vi "SaveFiles.vi"(0 "Refnum in":refnum<k34>, 1 "Analyte":string, 2 "fileCreateTime":timestamp, 4 "Array 2":waveform(dbl)[](array[waveform]), 6 "ParameterValues":string[](array[string]), 8 "output path":path, 10 "ParameterNames":string[](array[string])) -> (14 "Refnum out":refnum<k34>, 15 "seconds since 1Jan1904":timestamp)   [LabVIEW 2024]
panel:
  out "error out":errorcluster
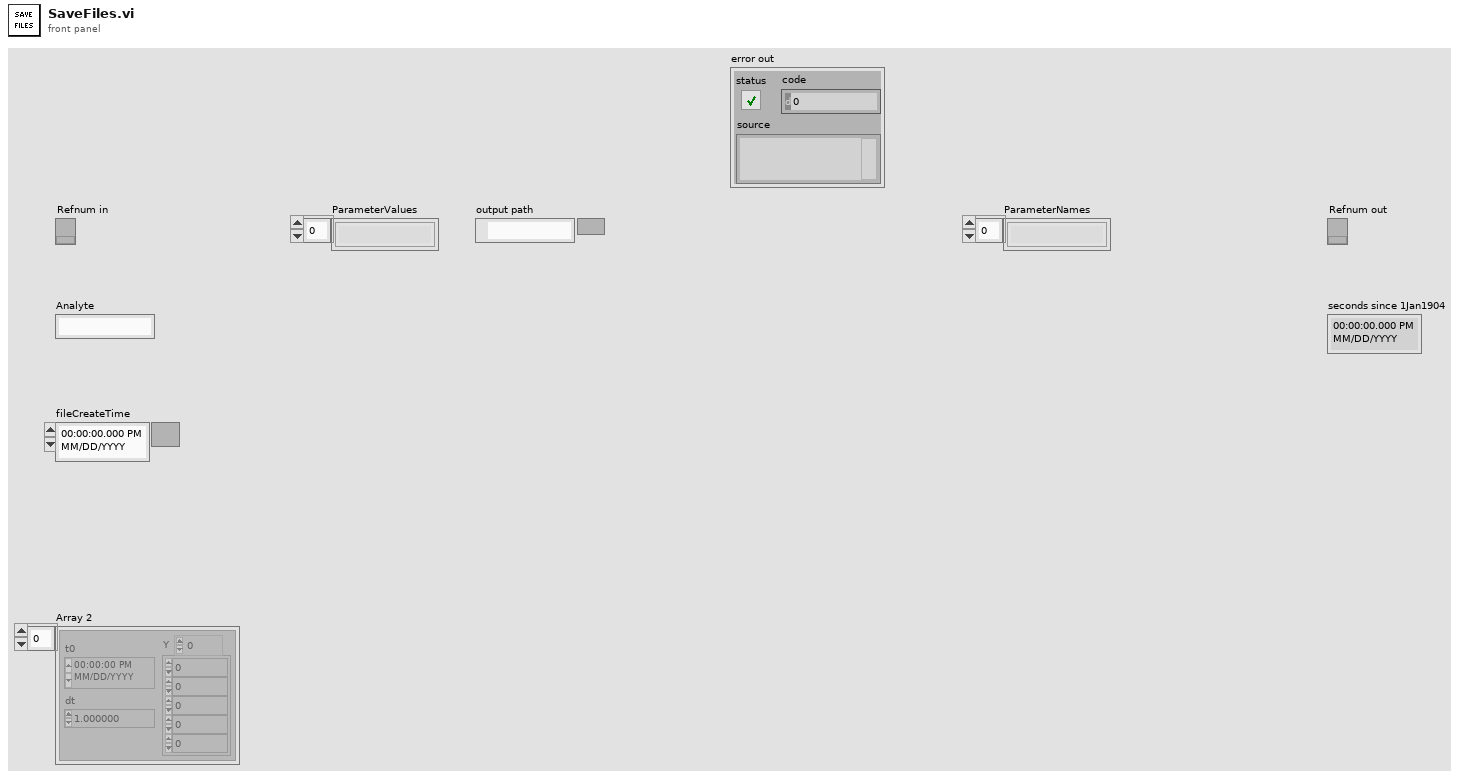
[diagram p1: front panel]
types:
  T1 = enum16{"open", "open or create", "create or replace", "create", "open (read-only)"}
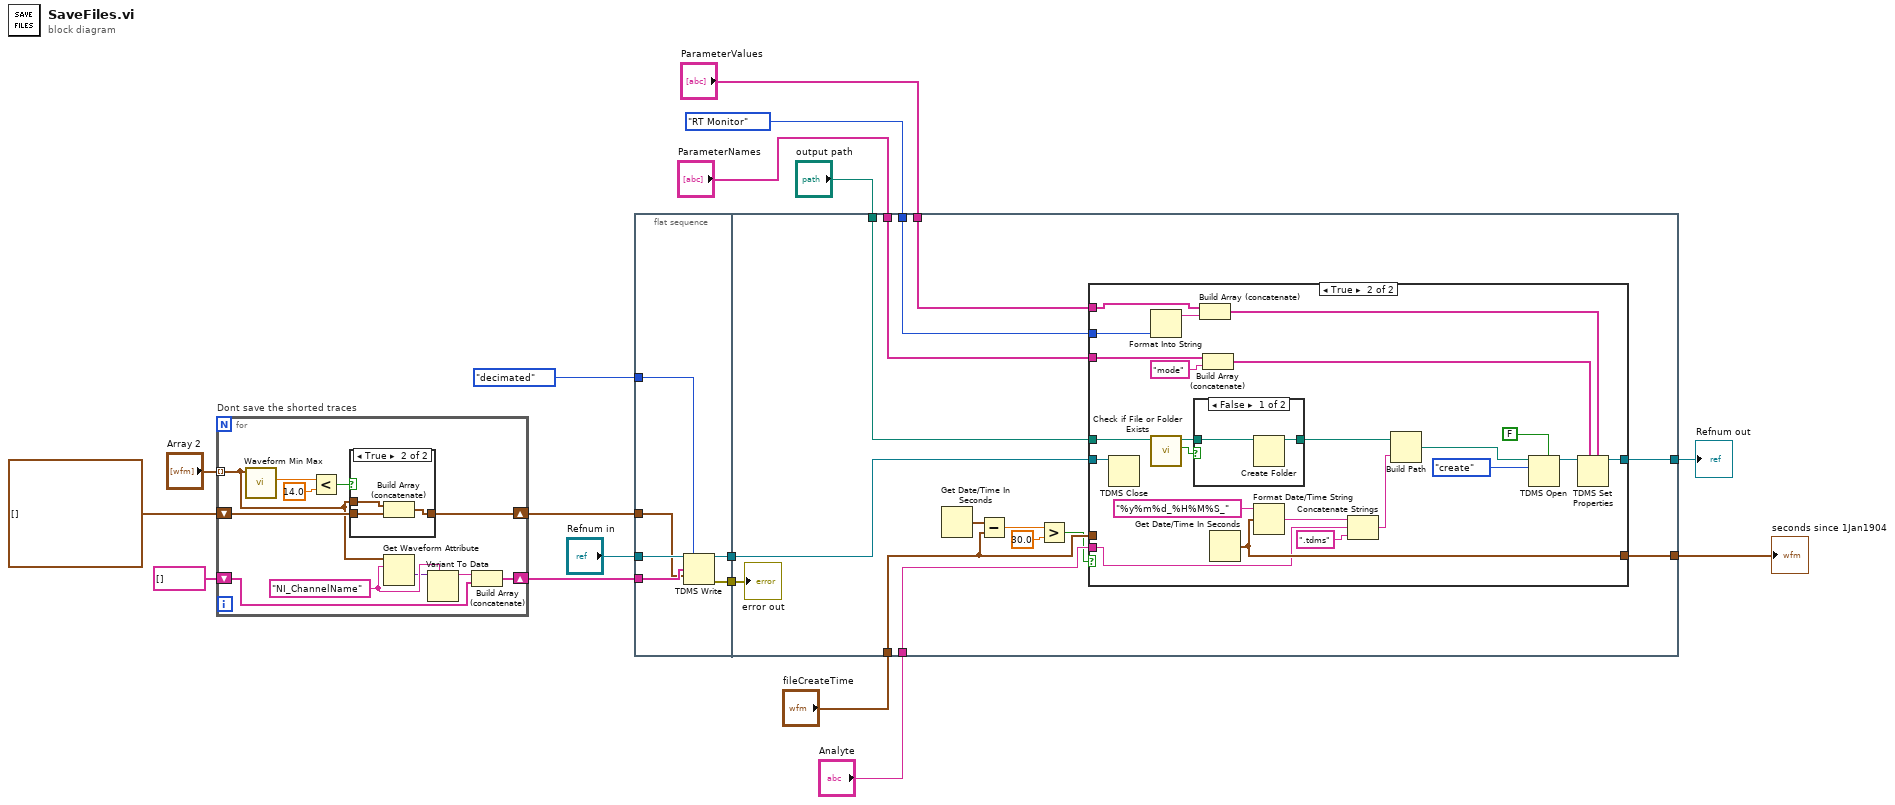
[diagram p0: block diagram]
diagram:
  n1 = for "Dont save the shorted traces" {
    tunnel: "Array 2" -> [w19] mode=indexing
    shift-right: [w25] -> w10
    shift-left: waveform(dbl)[] [] -> [w26]
    shift-right: [w24] -> w9
    shift-left: string[] [] -> [w23]
    w22 = "NI_ChannelName" ("name")
    n2 = call <vilib>:"Waveform Min Max.vi"("waveform in"=w19) -> ("Y max"=w18:dbl)  [unwired: 5 in, 5 out]
    n3 = Less?(x=w18, y=14.0) -> (x < y?=w27:bool)
    n4 = case shown="True" w27 {
      tunnel: w19 -> [_ w32]
      tunnel: [w29 w31] -> w25
      tunnel: w26 -> [w29 w30]
      frame False {
      }
      frame True {
        n5 = Build Array (concatenate)(w32, w30) -> (w31:waveform(dbl)[])
      }
    }
    n6 = Get Waveform Attribute(6:w22, 7:w19) -> (1:w20:variant)  [unwired: 2 in, 3 out]
    n7 = Variant To Data(type=w22, Variant=w20) -> (data=w21:string)  [unwired: 1 in, 1 out]
    n8 = Build Array (concatenate)(w21, w23) -> (w24:string[])
  }
  n9 = flat-sequence {
    tunnel: "Refnum in" -> [w38]
    tunnel: enum16{"decimated", "interleaved"}."decimated" ("data layout (0:decimated)") -> [w37]
    tunnel: w9 -> [w36]
    tunnel: w10 -> [w35]
    tunnel: [w34] -> w2
    tunnel: [w33] -> w1
    tunnel: w2 -> [w52]
    tunnel: enum32{"RT Monitor", "IV Monitor"}."RT Monitor" ("Value") -> [w51]
    tunnel: [w50] -> w11
    tunnel: [w49] -> w12
    tunnel: "fileCreateTime" -> [w44]
    tunnel: "output path" -> [w48]
    tunnel: "ParameterNames" -> [w47]
    tunnel: "ParameterValues" -> [w46]
    tunnel: "Analyte" -> [w45]
    tunnel: w1 -> [w39]
    frame #0 {
      n10 = TDMS Write(0:w38, 1:w37, 7:w36, 9:w35) -> (4:w34:refnum<k34>, 15:w33:errorcluster)  [unwired: 2 in, 2 out]
    }
    frame #1 {
      n11 = Get Date/Time In Seconds() -> (seconds since 1Jan1904=w42:timestamp)
      n12 = Subtract(x=w42, y=w44) -> (x-y=w43:dbl)
      n13 = Greater?(x=w43, y=30.0) -> (0:w40:bool)
      n14 = case shown="True" w40 {
        tunnel: w52 -> [w54 w63]
        tunnel: w51 -> [_ w62]
        tunnel: [w54 w60] -> w50
        tunnel: [w53 w59] -> w49
        tunnel: w48 -> [_ w58]
        tunnel: w47 -> [_ w57]
        tunnel: w46 -> [_ w56]
        tunnel: w45 -> [_ w55]
        tunnel: w44 -> [w53 _]
        frame False {
        }
        frame True {
          n15 = TDMS Close(11:w63) -> ()  [unwired: 1 in, 2 out]
          n16 = Format Into String(w62) -> (resulting string=w61:string)  [unwired: 3 in, 1 out]
          n17 = call <vilib>:"Check if File or Folder Exists.vi"("path"=w58) -> ("file or folder exists?"=w77:bool, "dup path"=w72:path)  [unwired: 8 in, 1 out]
          n18 = case shown="False" w77 {
            tunnel: w72 -> [w79 w80]
            tunnel: [w78 w80] -> w73
            frame False {
              n19 = Create Folder(path (use dialog)=w79) -> (created path=w78:path)  [unwired: 2 in, 2 out]
            }
            frame True {
            }
          }
          n20 = Build Array (concatenate)(w56, w61) -> (w65:string[])
          n21 = Build Array (concatenate)(w57, "mode") -> (w64:string[])
          n22 = Get Date/Time In Seconds() -> (seconds since 1Jan1904=w59:timestamp)
          n23 = Format Date/Time String(time format string (%c)="%y%m%d_%H%M%S_", seconds (now)=w59) -> (date/time string=w68:string)  [unwired: 1 in]
          n24 = Concatenate Strings(w68, w55, ".tdms" ("string")) -> (w67:string)
          n25 = Build Path(base path=w73, name or relative path=w67) -> (appended path=w71:path)
          n26 = TDMS Open(5:FALSE ("create index file? (T)"), 10:T1."create" ("operation (0:open)"), 11:w71) -> (3:w76:refnum<k34>)  [unwired: 4 in, 1 out]
          n27 = TDMS Set Properties(5:w65, 7:w64, 11:w76) -> (3:w60:refnum<k34>)  [unwired: 3 in, 3 out]
        }
      }
      "error out" <- w39
    }
  }
  "seconds since 1Jan1904" <- w12
  "Refnum out" <- w11
